vi "Put.vi"() -> ()   [LabVIEW 2010]
uses:
  <userlib>/caLab/sub/caLabPut42.vi
panel:
  out "Value History":dbl(graph)
  out "Value":dbl(knob) scale=0.0..10.0
  in  "stop":bool
  in  "Process Variable":string caption="Process Variable to Write To (Numeric Only)"
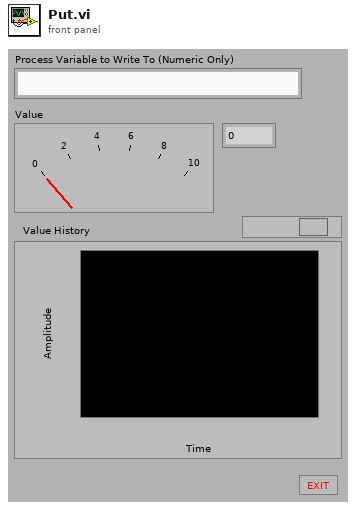
[diagram p1: front panel]
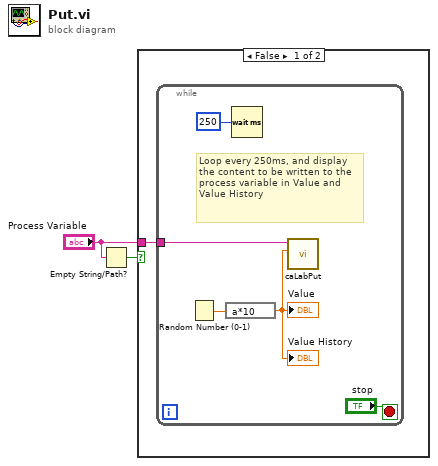
[diagram p0: block diagram]
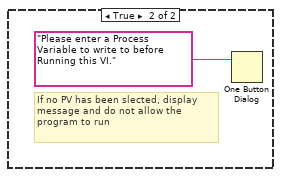
[diagram p2: hidden frame]
diagram:
  n1 = Empty String/Path?(string/path="Process Variable") -> (empty?=w1:bool)
  n2 = case shown="False" w1 {
    tunnel: "Process Variable" -> [w3 _]
    frame False {
      n3 = while {
        tunnel: w3 -> [w8]
        stop <- "stop" stop-if-true
        # "Loop every 250ms, and display the content to be written to the process variable in Value and Value History"
        n4 = Random Number (0-1)() -> (number: 0 to 1=w5:dbl)
        n5 = expression code="a*10"(w5) -> (w4:dbl)
        "Value History" <- w4
        "Value" <- w4
        n6 = Wait (ms)(milliseconds to wait=u32 250) -> ()  [unwired: 1 out]
        n7 = call-poly <userlib>:"caLabPut.vi"("values"=w4, "PV name(s)"=w8) -> ()  [unwired: 6 in, 4 out]
      }
    }
    frame True {
      # "If no PV has been slected, display message and do not allow the program to run"
      n8 = One Button Dialog(message="Please enter a Process Variable to write to before Running this VI.") -> ()  [unwired: 1 in, 1 out]
    }
  }
